vi "Global Value 2.vi"(9 "Number of frames":i32, 10 "Samples per frame control":u32=262144, 11 "Max DRAM address":u32) -> ()   [LabVIEW 2015]
uses:
  <vilib>/rvi/Emulation/niFpgaSctlEmulationGetInTimedLoop.vi
  Globals/Global_Sample per Frame.vi
  <vilib>/rvi/Emulation/niFpgaProcessEmulError.vi
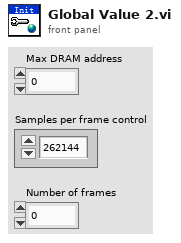
[diagram p1: front panel]
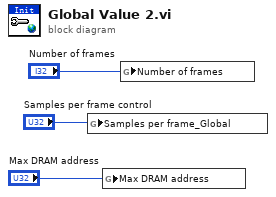
[diagram p0: block diagram]
diagram:
  n1 = global write "Global_Sample per Frame.vi" "Samples per frame_Global"("Samples per frame control") -> ()
  n2 = global write "Global_Sample per Frame.vi" "Max DRAM address"("Max DRAM address") -> ()
  n3 = global write "Global_Sample per Frame.vi" "Number of frames"("Number of frames") -> ()
